vi "PrepareWaveformDataForTDMS.vi"(8 "error in (no error)":errorcluster, 11 "WaveformArray in":waveform(dbl)[](array[waveform])) -> (0 "error out":errorcluster, 1 "Measurement Data":dbl[][](array[numeric]), 2 "Channel Names":string[](array[string]), 3 "TimeStamp":timestamp)   [LabVIEW 2018, in "Visualization.lvlib" / "VisualizeSensor.lvclass"]
uses:
  VisualizeSensor.lvclass
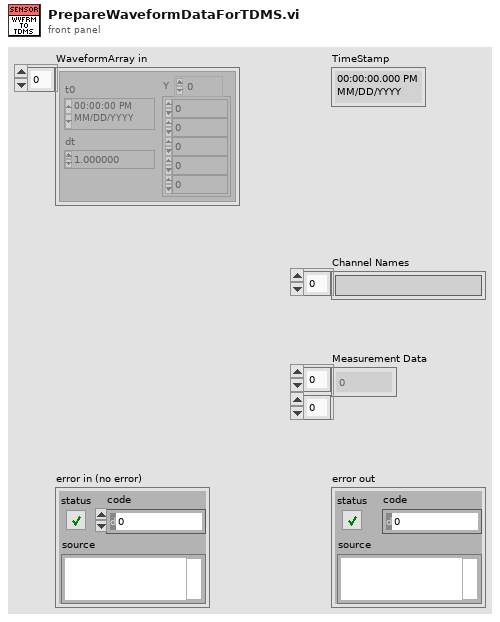
[diagram p1: front panel]
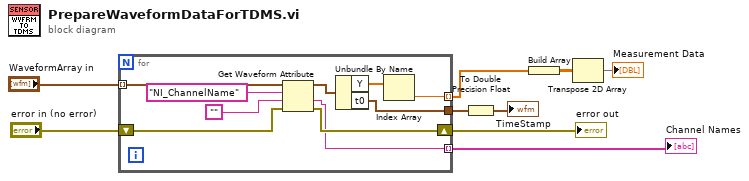
[diagram p0: block diagram]
diagram:
  n1 = for {
    tunnel: "WaveformArray in" -> [w18] mode=indexing
    tunnel: [w13] -> w7
    tunnel: [w12] -> w4 mode=indexing
    shift-right: [w10] -> w5
    shift-left: "error in (no error)" -> [w11]
    tunnel: [w9] -> w3 mode=indexing
    n2 = Get Waveform Attribute(4:w11, 5:"", 6:"NI_ChannelName" ("name"), 7:w18) -> (0:w10:errorcluster, 1:w9:string, 3:w15:waveform(dbl))  [unwired: 1 out]
    n3 = Unbundle By Name(w15) -> ("Y"=w14:dbl[], "t0"=w13:timestamp)
    n4 = Index Array(array=w14) -> (element=w12:dbl)  [unwired: 1 in]
  }
  "error out" <- w5
  "Channel Names" <- w3
  "TimeStamp" <- w7
  n5 = To Double Precision Float(number=w7) -> ()  [unwired: 1 out]
  n6 = Build Array(w4) -> (w2:dbl[][])
  n7 = Transpose 2D Array(2D array=w2) -> (transposed array=→"Measurement Data":dbl[][])
